vi "TrivialTop.vi"() -> ()   [LabVIEW 2010]
panel:
  in  "Combo Box":string(combo)
  out "Tank":dbl(slide) scale=0.0..10.0
  in  "Slide":dbl(slide) scale=0.0..10.0
  in  "Numeric":dbl
  # "Text box made in trunk  version"
  # "Another trunk text box"
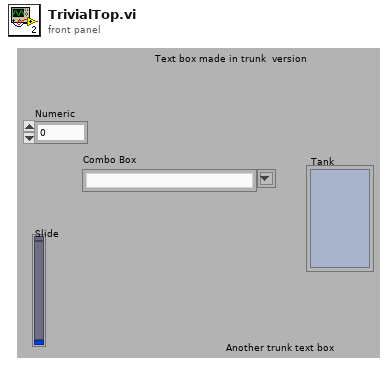
[diagram p1: front panel]
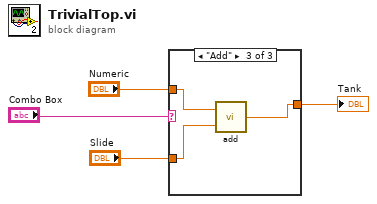
[diagram p0: block diagram]
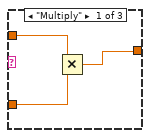
[diagram p2: hidden frame]
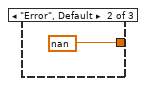
[diagram p3: hidden frame]
diagram:
  n1 = case shown="\"Add\"" "Combo Box" {
    tunnel: [w5 nan w9] -> w3
    tunnel: "Numeric" -> [w7 _ w11]
    tunnel: "Slide" -> [w6 _ w10]
    frame "Multiply" {
      n2 = Multiply(x=w7, y=w6) -> (x*y=w5:dbl)
    }
    frame "Error", Default {
    }
    frame "Add" {
      n3 = call "add.vi"("Slide"=w10, "Numeric 2"=w11) -> ("Numeric"=w9:dbl)
    }
  }
  "Tank" <- w3
